vi "EJERCICIO-5-2C.vi"(11 "Array":string[][](array[string])) -> (3 "spreadsheet string":string)   [LabVIEW 2017]
panel:
  out "Error Out":errorcluster
  in  "Error In":errorcluster
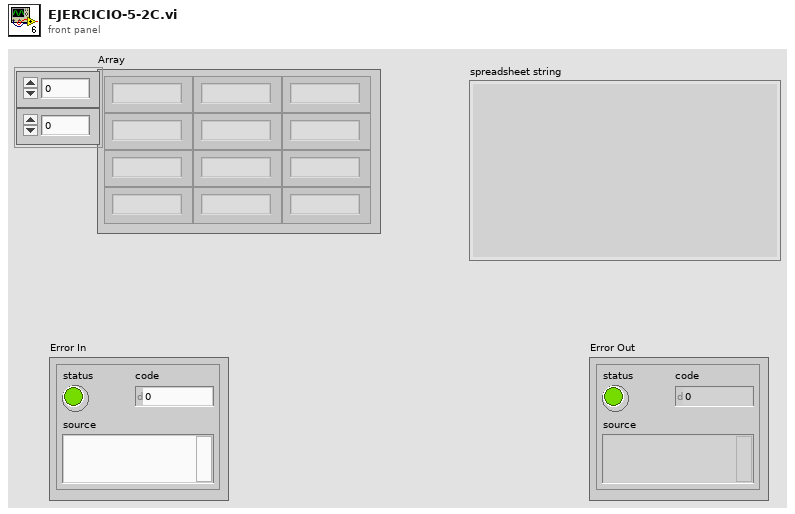
[diagram p1: front panel]
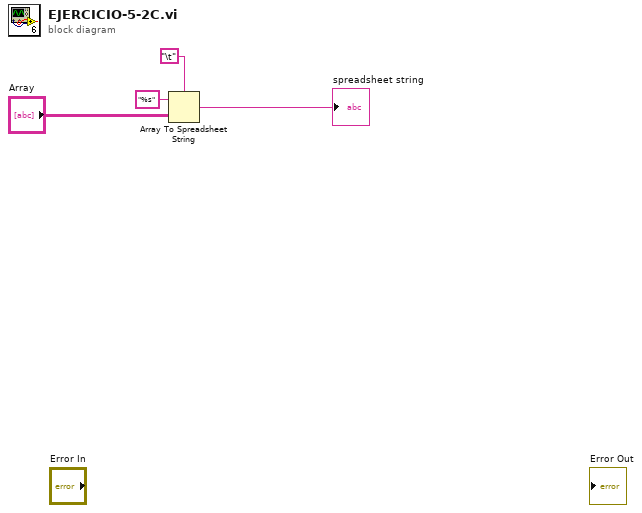
[diagram p0: block diagram]
diagram:
  n1 = Array To Spreadsheet String(delimiter (Tab)="\t", array="Array", 3:"%s" ("format string")) -> (spreadsheet string=→"spreadsheet string":string)
